vi "Return Default Object.vi"(10 "Object":refnum<class>) -> (2 "Default Object Instance":refnum<class>)   [LabVIEW 2021, in "jettl.lvlib"]
uses:
  jettl.lvlib
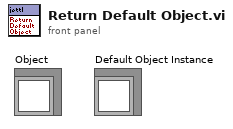
[diagram p1: front panel]
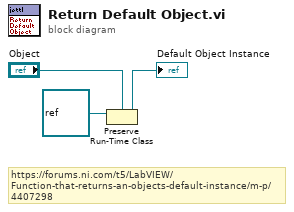
[diagram p0: block diagram]
diagram:
  # "https://forums.ni.com/t5/LabVIEW/Function-that-returns-an-objects-default-instance/m-p/4407298"
  n1 = Preserve Run-Time Class(object in=refnum<class> refnum ("LabVIEW Object"), 2:"Object") -> (object out=→"Default Object Instance":refnum<class>)  [unwired: 1 in, 1 out]
